vi "Read Ratiometer file Full Data.vi"() -> ()   [LabVIEW 2013]
uses:
  Users/james.powell/RAL Isotope Ratiometer/Ratiometer/Slow DAQ Folder/Readings.ctl
  Users/james.powell/RAL Isotope Ratiometer/Ratiometer Fitting/Fitting Model/Etalon Cal.ctl
  Users/james.powell/RAL Isotope Ratiometer/Ratiometer/Support/IsotopeData.ctl
  Users/james.powell/RAL Isotope Ratiometer/Ratiometer/Support/LaserData.ctl
  JSONtext.lvlib
  <vilib>/addons/JSON API/Get Polymorphic/JSON GetSet.lvlib
  <vilib>/addons/JSON API/JSON Value/Set from JSON string.vi
  <vilib>/addons/JSON API/JSON Value/JSON Value.lvclass
  <vilib>/addons/JSON API/Variant JSON/Get as Variant.vi
  <vilib>/addons/JSON API/Variant JSON/Variant JSON.lvlib
panel:
  out "data":T5
  out "time":dbl[](array[numeric]) format="%#_3p"
  out "Time":dbl format="%#_3p"
  out "Variant out":variant
  out "error out":errorcluster
  out "text":string
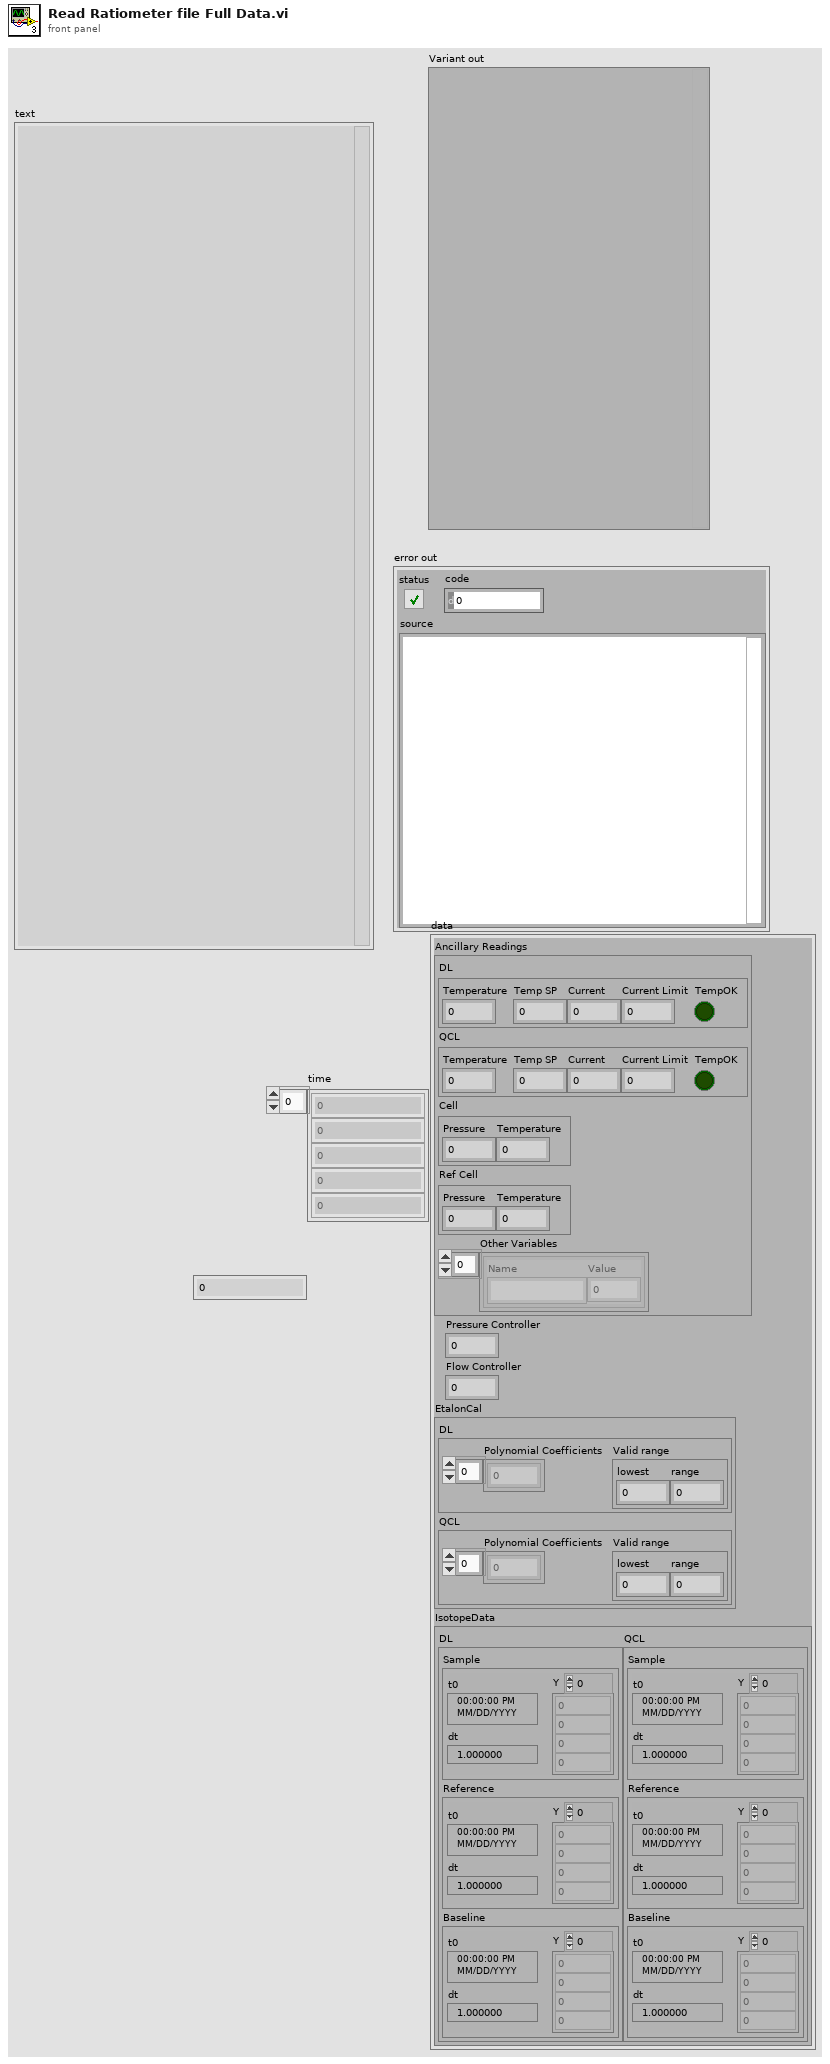
[diagram p1: front panel]
types:
  T1 = typedef "Readings.ctl" = cluster{"DL":cluster{"Temperature":dbl, "Temp SP":dbl, "Current":dbl, "Current Limit":dbl, "TempOK":bool}, "QCL":cluster{"Temperature":dbl, "Temp SP":dbl, "Current":dbl, "Current Limit":dbl, "TempOK":bool}, "Cell":cluster{"Pressure":dbl, "Temperature":dbl}, "Ref Cell":cluster{"Pressure":dbl, "Temperature":dbl}, "Other Variables":cluster{"Name":string, "Value":dbl}[]}
  T2 = typedef "Etalon Cal.ctl" = cluster{"DL":cluster{"Polynomial Coefficients":dbl[], "Valid range":cluster{"lowest":i32, "range":i32}}, "QCL":cluster{"Polynomial Coefficients":dbl[], "Valid range":cluster{"lowest":i32, "range":i32}}}
  T3 = typedef "IsotopeData.ctl" = cluster{"DL":T4, "QCL":T4}
  T4 = typedef "LaserData.ctl" = cluster{"Sample":waveform(dbl), "Reference":waveform(dbl), "Baseline":waveform(dbl)}
  T5 = cluster{"Ancillary Readings":T1, "Pressure Controller":sgl, "Flow Controller":sgl, "EtalonCal":T2, "IsotopeData":T3}
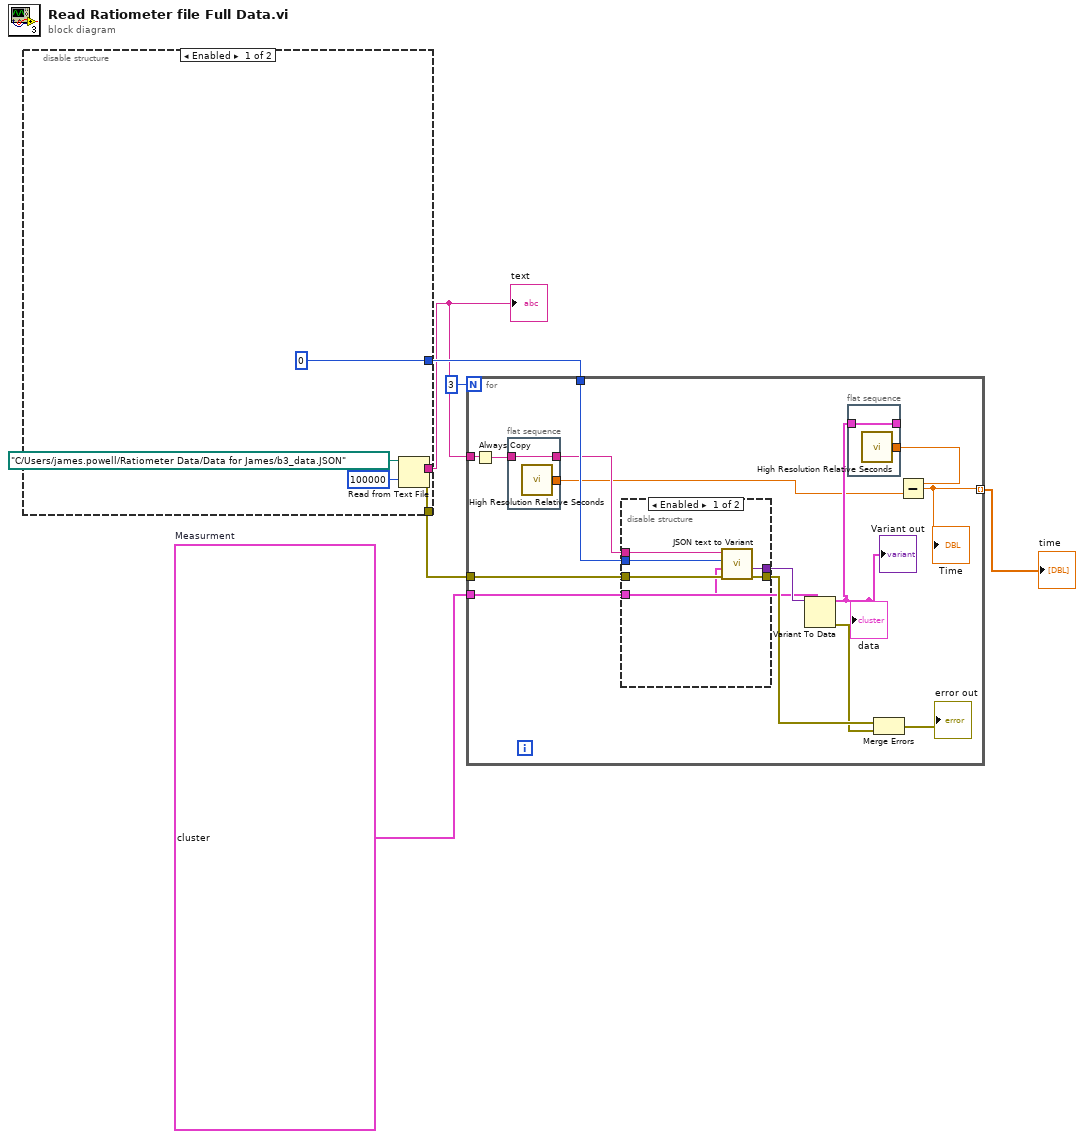
[diagram p0: block diagram]
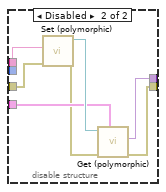
[diagram p2: hidden frame]
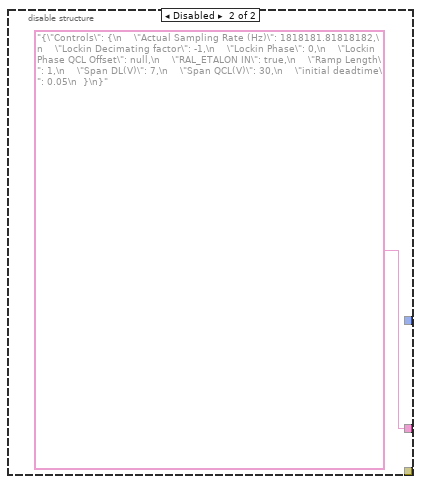
[diagram p3: hidden frame]
diagram:
  w4 = T5 {"Ancillary Readings"={"DL"={"Temperature"=nan, "Temp SP"=nan, "Current"=nan, "Current Limit"=nan, "TempOK"=FALSE}, "QCL"={"Temperature"=nan, "Temp SP"=nan, "Current"=nan, "Current Limit"=nan, "TempOK"=FALSE}, "Cell"={"Pressure"=nan, "Temperature"=nan}, "Ref Cell"={"Pressure"=nan, "Temperature"=nan}, "Other Variables"=[]}, "Pressure Controller"=0.0, "Flow Controller"=1.0, "EtalonCal"={"DL"={"Polynomial Coefficients"=[], "Valid range"={"lowest"=0, "range"=0}}, "QCL"={"Polynomial Coefficients"=[], "Valid range"={"lowest"=0, "range"=0}}}, "IsotopeData"={"DL"={"Sample"={"t0"=timestamp(0 s since 1904-01-01), "dt"=1.0, "Y"=[0.0, 0.0, 123.0, 0.0, 0.0, 123.0]}, "Reference"={"t0"=timestamp(0 s since 1904-01-01), "dt"=1.0, "Y"=[]}, "Baseline"={"t0"=timestamp(0 s since 1904-01-01), "dt"=0.0, "Y"=[]}}, "QCL"={"Sample"={"t0"=timestamp(0 s since 1904-01-01), "dt"=1.0, "Y"=[]}, "Reference"={"t0"=timestamp(0 s since 1904-01-01), "dt"=1.0, "Y"=[]}, "Baseline"={"t0"=timestamp(0 s since 1904-01-01), "dt"=0.0, "Y"=[]}}}}  # Measurment
  n1 = disable-structure shown="Enabled" {
    disable-tunnel: [w10 "{\"Controls\": {\n    \"Actual Sampling Rate (Hz)\": 1818181.81818182,\n    \"Lockin Decimating factor\": -1,\n    \"Lockin Phase\": 0,\n    \"Lockin Phase QCL Offset\": null,\n    \"RAL_ETALON IN\": true,\n    \"Ramp Length\": 1,\n    \"Span DL(V)\": 7,\n    \"Span QCL(V)\": 30,\n    \"initial deadtime\": 0.05\n  }\n}" ("text")] -> w3
    disable-tunnel: [w9 _] -> w6
    disable-tunnel: [0 ("Offset") _] -> w5
    frame Enabled {
      n2 = Read from Text File(file (use dialog)=path "C:/Users/james.powell/Ratiometer Data/Data for James/b3_data.JSON", count=100000) -> (text=w10:string, error out=w9:errorcluster)  [unwired: 2 in, 2 out]
    }
    frame Disabled {
    }
  }
  "text" <- w3
  n3 = for {
    N: 3 -> [_]
    tunnel: w6 -> [w25]
    tunnel: w5 -> [w24]
    tunnel: w4 -> [w20]
    tunnel: w3 -> [w18]
    tunnel: [w14] -> w2 mode=indexing
    n4 = Always Copy(1:w18) -> (0:w13:string)
    n5 = flat-sequence {
      tunnel: [w43] -> w19
      tunnel: w13 -> [w43]
      tunnel: [w42] -> w16
      frame #0 {
        n6 = call <vilib>:"High Resolution Relative Seconds.vi"() -> ("relative seconds"=w42:dbl)
      }
    }
    n7 = disable-structure shown="Enabled" {
      disable-tunnel: [w32 w36] -> w26
      disable-tunnel: w25 -> [w31 w33]
      disable-tunnel: w24 -> [w30 _]
      disable-tunnel: [w29 w35] -> w23
      disable-tunnel: w20 -> [w28 w37]
      disable-tunnel: w19 -> [w27 w39]
      frame Enabled {
        n8 = call "JSON text to Variant.vi"("error in (no error)"=w31, "Variant (Data Type)"=w28, "Offset"=w30, "JSON"=w27) -> ("error out"=w29:errorcluster, "Variant out"=w32:variant)  [unwired: 6 in]
      }
      frame Disabled {
        n9 = call-poly <vilib>:"Set (polymorphic).vi"("error in (no error)"=w33, "JSON stream"=w39) -> ("error out"=w34:errorcluster, "JSON Value out"=w38:refnum<class "JSON Value.lvclass">)  [unwired: 7 in, 1 out]
        n10 = call-poly <vilib>:"Get (polymorphic).vi"("Variant (Data Type)"=w37, "error in (no error)"=w34, "JSON in"=w38) -> ("error out"=w35:errorcluster, "Variant out"=w36:variant)  [unwired: 6 in, 1 out]
      }
    }
    n11 = Variant To Data(type=w20, Variant=w26) -> (data=w17:T5, error out=w21:errorcluster)  [unwired: 1 in]
    "Variant out" <- w17
    "data" <- w17
    n12 = flat-sequence {
      tunnel: [w41] -> _
      tunnel: w17 -> [w41]
      tunnel: [w40] -> w15
      frame #0 {
        n13 = call <vilib>:"High Resolution Relative Seconds.vi"() -> ("relative seconds"=w40:dbl)
      }
    }
    n14 = Merge Errors(w23, w21) -> (→"error out":errorcluster)
    n15 = Subtract(x=w15, y=w16) -> (x-y=w14:dbl)
    "Time" <- w14
  }
  "time" <- w2
